vi "Flattened Path to Path.vi"(10 "Flattened Path String":string) -> (2 "path":path)   [LabVIEW 2013, in "OpenConvert.lvlib"]
uses:
  OpenConvert.lvlib
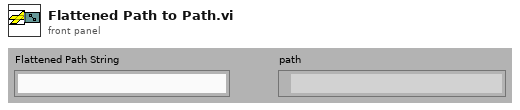
[diagram p1: front panel]
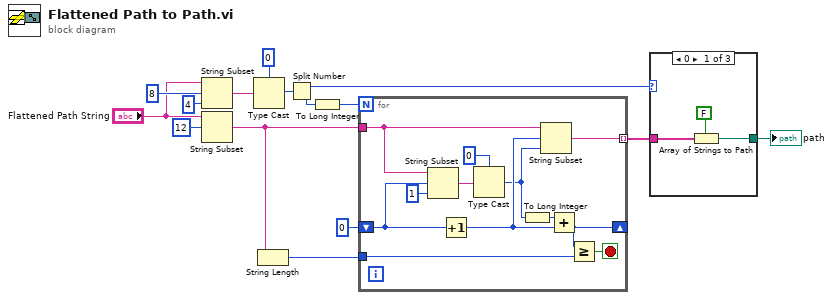
[diagram p0: block diagram]
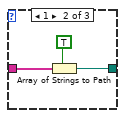
[diagram p2: hidden frame]
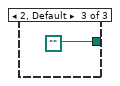
[diagram p3: hidden frame]
diagram:
  n1 = String Subset(string="Flattened Path String", offset (0)=8, length (rest)=4 ("offset (0)")) -> (substring=w13:string)
  n2 = String Subset(string="Flattened Path String", offset (0)=12) -> (substring=w2:string)  [unwired: 1 in]
  n3 = Type Cast(type=u32 0, x=w13) -> (*(type *) &x=w7:u32)
  n4 = String Length(string=w2) -> (length=w1:i32)
  n5 = Split Number(x=w7) -> (hi(x)=w5:u16, lo(x)=w3:u16)
  n6 = To Long Integer(number=w3) -> (32bit integer=w4:i32)
  n7 = for {
    N: w4 -> [_]
    tunnel: w2 -> [w23]
    shift-right: [w16] -> _
    shift-left: 0 -> [w26]
    tunnel: [w20] -> w9 mode=indexing
    tunnel: w1 -> [w17]
    stop <- w18 stop-if-true
    n8 = String Subset(string=w23, offset (0)=w26, length (rest)=1 ("length (rest)")) -> (substring=w25:string)
    n9 = Increment(x=w26) -> (x+1=w22:i32)
    n10 = Type Cast(type=u8 0, x=w25) -> (*(type *) &x=w21:u8)
    n11 = To Long Integer(number=w21) -> (32bit integer=w19:i32)
    n12 = String Subset(string=w23, offset (0)=w22, length (rest)=w21) -> (substring=w20:string)
    n13 = Add(x=w19, y=w22) -> (x+y=w16:i32)
    n14 = Greater Or Equal?(x=w16, y=w17) -> (x >= y?=w18:bool)
  }
  n15 = case shown="0" w5 {
    tunnel: w9 -> [w30 w33 _]
    tunnel: [w29 w32 path ""] -> w8
    frame 0 {
      n16 = Array of Strings to Path(0:w30, 1:FALSE ("relative")) -> (2:w29:path)
    }
    frame 1 {
      n17 = Array of Strings to Path(0:w33, 1:TRUE ("relative")) -> (2:w32:path)
    }
    frame 2, Default {
    }
  }
  "path" <- w8
